vi "Caller-RegisterForMessageSpecificType.vi"(8 "error in (no error)":errorcluster, 9 "_Msg-Filter":refnum<class "_Msg-Filter.lvclass">, 10 "MailBoxMessage":refnum<class "MailBoxMessage.lvclass">, 11 "MailboxClient in":refnum<class "MailboxClient.lvclass">) -> (0 "error out":errorcluster, 3 "MailboxClient out":refnum<class "MailboxClient.lvclass">)   [LabVIEW 2020, in "MailboxClient.lvlib" / "MailboxClient.lvclass"]
uses:
  MailboxClient.lvclass
  C:/Program Files (x86)/National Instruments/LabVIEW 2020/vi.lib/ActorFramework/Actor/Actor.lvclass
  <vilib>/ActorFramework/Actor/Actor.lvclass/Actor.ctl
  MailboxManager/MailboxManager Messages/RegisterForMessageSpecificType Msg/RegisterForMessageSpecificType Msg.lvclass/RegisterForMessageSpecificType Msg.ctl
  <vilib>/ActorFramework/Message Enqueuer/Message Enqueuer.lvclass/Message Enqueuer.ctl
  <vilib>/ActorFramework/Message Enqueuer/Enqueue.vi
  MailboxManager/MailboxManager Messages/RegisterForMessageSpecificType Msg/RegisterForMessageSpecificType Msg.lvclass
  C:/Program Files (x86)/National Instruments/LabVIEW 2020/vi.lib/ActorFramework/Message/Message.lvclass
  <vilib>/ActorFramework/Message Priority Queue/Priority Enqueue.vi
  <vilib>/ActorFramework/Actor/Actor.lvclass
  C:/Users/taylo/Projects/LabVIEW/ActorMailbox/MailboxClient/MailboxClient/MailboxClient.lvclass
  MailboxManager/_Msg-Filter/_Msg-Filter.lvclass
  MailboxManager/MailBoxMessage/MailBoxMessage.lvclass
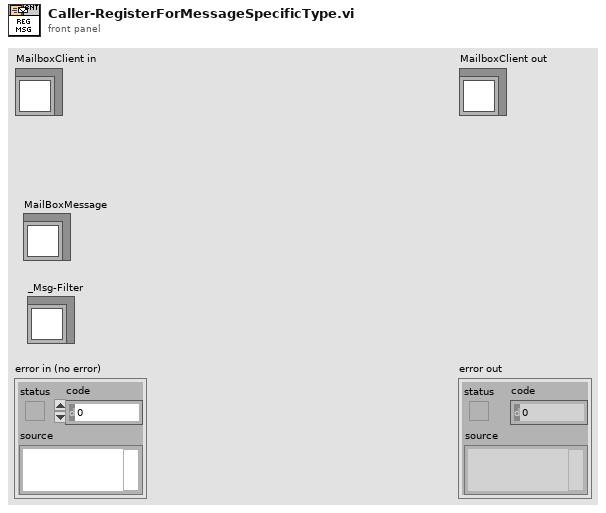
[diagram p1: front panel]
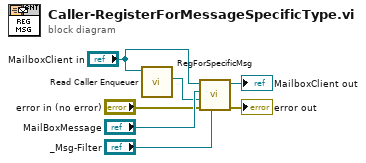
[diagram p0: block diagram]
diagram:
  n1 = call <vilib>:"Read Caller Enqueuer.vi"("Actor"="MailboxClient in") -> ("Caller Enqueuer"=w6:refnum<class "Message Enqueuer.lvclass">)  [unwired: 10 in]
  n2 = call-dynamic "RegForSpecificMsg.vi"("_Msg-Filter"="_Msg-Filter", "error in (no error)"="error in (no error)", "MailboxManager"=w6, "MailBoxMessage"="MailBoxMessage", "MailboxClient in"="MailboxClient in") -> ("error out"=→"error out":errorcluster, "MailboxClient out"=→"MailboxClient out":refnum<class "MailboxClient.lvclass">)  [unwired: 5 in]
